vi "B7_72.vi"(4 "error in":T13, 7 "Command":T14) -> (0 "error out":T13, 3 "Response":T11)   [LabVIEW 2018]
uses:
  MOKO_LabViewLibrary/MokoLowLevel/MokoLowLovelControl/MLLC_Command.ctl
  MOKO_LabViewLibrary/MokoLowLevel/MokoLowLovelControl/MLLC_Error.ctl
  MOKO_LabViewLibrary/MokoLowLevel/MokoLowLovelControl/MLLC_Mode.ctl
  MOKO_LabViewLibrary/MokoLowLevel/MokoLowLovelControl/MLLC_Response.ctl
  MOKO_LabViewLibrary/MokoLowLevel/MokoLowLovelControl/MLLC_DriverName.ctl
  MOKO_LabViewLibrary/MokoLowLevel/MokoLowLovelControl/MLLC_ResponseInit.ctl
  MOKO_LabViewLibrary/MokoLowLevel/MokoLowLovelControl/MLLC_Request.ctl
  MOKO_LabViewLibrary/MokoLowLevel/MokoLowLovelControl/MLLC_ErrorCode.ctl
  MOKO_LabViewLibrary/MokoLowLevel/MokoLowLovelControl/MLLC_ConnectCluster.ctl
  MOKO_LabViewLibrary/MokoLowLevel/MokoLowLovelControl/MLLC_InterfaceType.ctl
  MOKO_LabViewLibrary/MokoLowLevel/MokoLowLovelControl/MLLC_OpenedSession.ctl
  MOKO_LabViewLibrary/MokoLowLevel/MokoLowLovelControl/MLLC_InterfaceSettings.ctl
  MOKO_LabViewLibrary/MokoLowLevel/MokoLowLovelControl/MLLC_InterfaceKind.ctl
  MOKO_LabViewLibrary/MokoLowLevel/MokoLowLovelControl/MLLC_Rs232Settings.ctl
panel:
  in  "Settings":T7={"Data"={"Connect"={"InterfaceType"=enum."VISA", "OpenedSession"="COM1", "InterfaceSettings"={"Interface"=enum."RS232", "EOS 4 read"=enum."LF (\\n)", "EOS 4 write"=enum."LF (\\n)", "TMO, ms"=10000, "Sett"=variant(cluster{"Baud Rate":u32, "Data Bits":u16, "Parity":u16, "Stop Bits":u16, "Flow Control":u16, "Eho":bool} {"Baud Rate"=75, "Data Bits"=0, "Parity"=0, "Stop Bits"=0, "Flow Control"=0, "Eho"=FALSE})}}, "Delay, ms"=100, "Function"=enum."VDC"}, "Saved Data"=variant}
  in  "Error Code":T6=5422
  in  "Request":T8="B2"
  in  "ResponseInit":T9="U4G1A0"
  in  "Driver Name":T10="B7_72"
  in  "Mode":T12=enum."Check"
  # "B7-72"
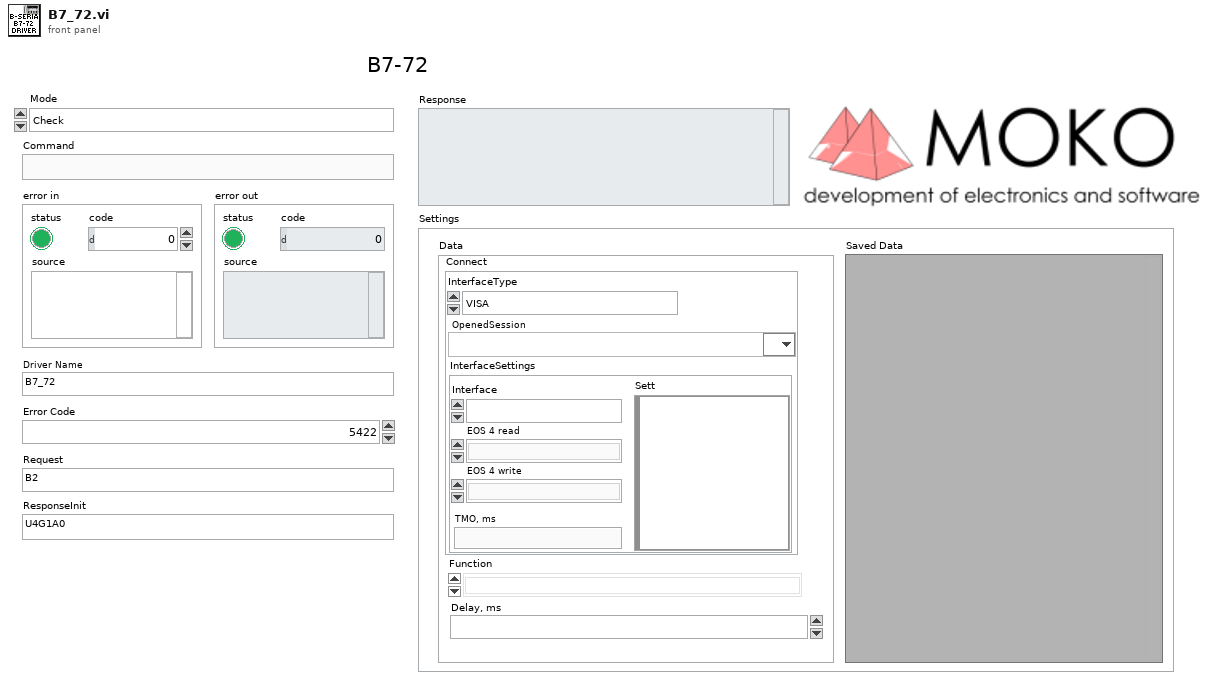
[diagram p1: front panel]
types:
  T1 = typedef "MLLC_ConnectCluster.ctl" = cluster{"InterfaceType":T2, "OpenedSession":T3, "InterfaceSettings":T4}
  T2 = typedef "MLLC_InterfaceType.ctl" = enum16{"VISA", "Prologix USB-GPIB"}
  T3 = typedef "MLLC_OpenedSession.ctl" = refnum<visa-resource-name>
  T4 = typedef "MLLC_InterfaceSettings.ctl" = cluster{"Interface":T5, "EOS 4 read":enum16{"Default (=EOS 4 write)", "CR (\\r)", "LF (\\n)", "None"}, "EOS 4 write":enum16{"CR+LF (\\r\\n)", "CR (\\r)", "LF (\\n)", "None"}, "TMO, ms":i32, "Sett":variant}
  T5 = typedef "MLLC_InterfaceKind.ctl" = enum16{"RS232", "GPIB", "USB", "Ethernet", "another"}
  T6 = typedef "MLLC_ErrorCode.ctl" = u32
  T7 = cluster{"Data":cluster{"Connect":T1, "Delay, ms":T6, "Function":enum16{"F", "T", "R4", "R", "IAC", "IDC", "VAC", "VDC"}}, "Saved Data":variant}
  T8 = typedef "MLLC_Request.ctl" = string
  T9 = typedef "MLLC_ResponseInit.ctl" = string
  T10 = typedef "MLLC_DriverName.ctl" = string
  T11 = typedef "MLLC_Response.ctl" = string
  T12 = typedef "MLLC_Mode.ctl" = enum16{"get", "set", "close", "Init", "Check"}
  T13 = typedef "MLLC_Error.ctl" = errorcluster
  T14 = typedef "MLLC_Command.ctl" = string
  T15 = cluster{"Connect":T1, "Delay, ms":T6, "Function":enum16{"F", "T", "R4", "R", "IAC", "IDC", "VAC", "VDC"}}
  T16 = enum16{"F", "T", "R4", "R", "IAC", "IDC", "VAC", "VDC"}
  T17 = typedef "MLLC_Rs232Settings.ctl" = cluster{"Baud Rate":u32, "Data Bits":u16, "Parity":u16, "Stop Bits":u16, "Flow Control":u16, "Eho":bool, "Address":dbl}
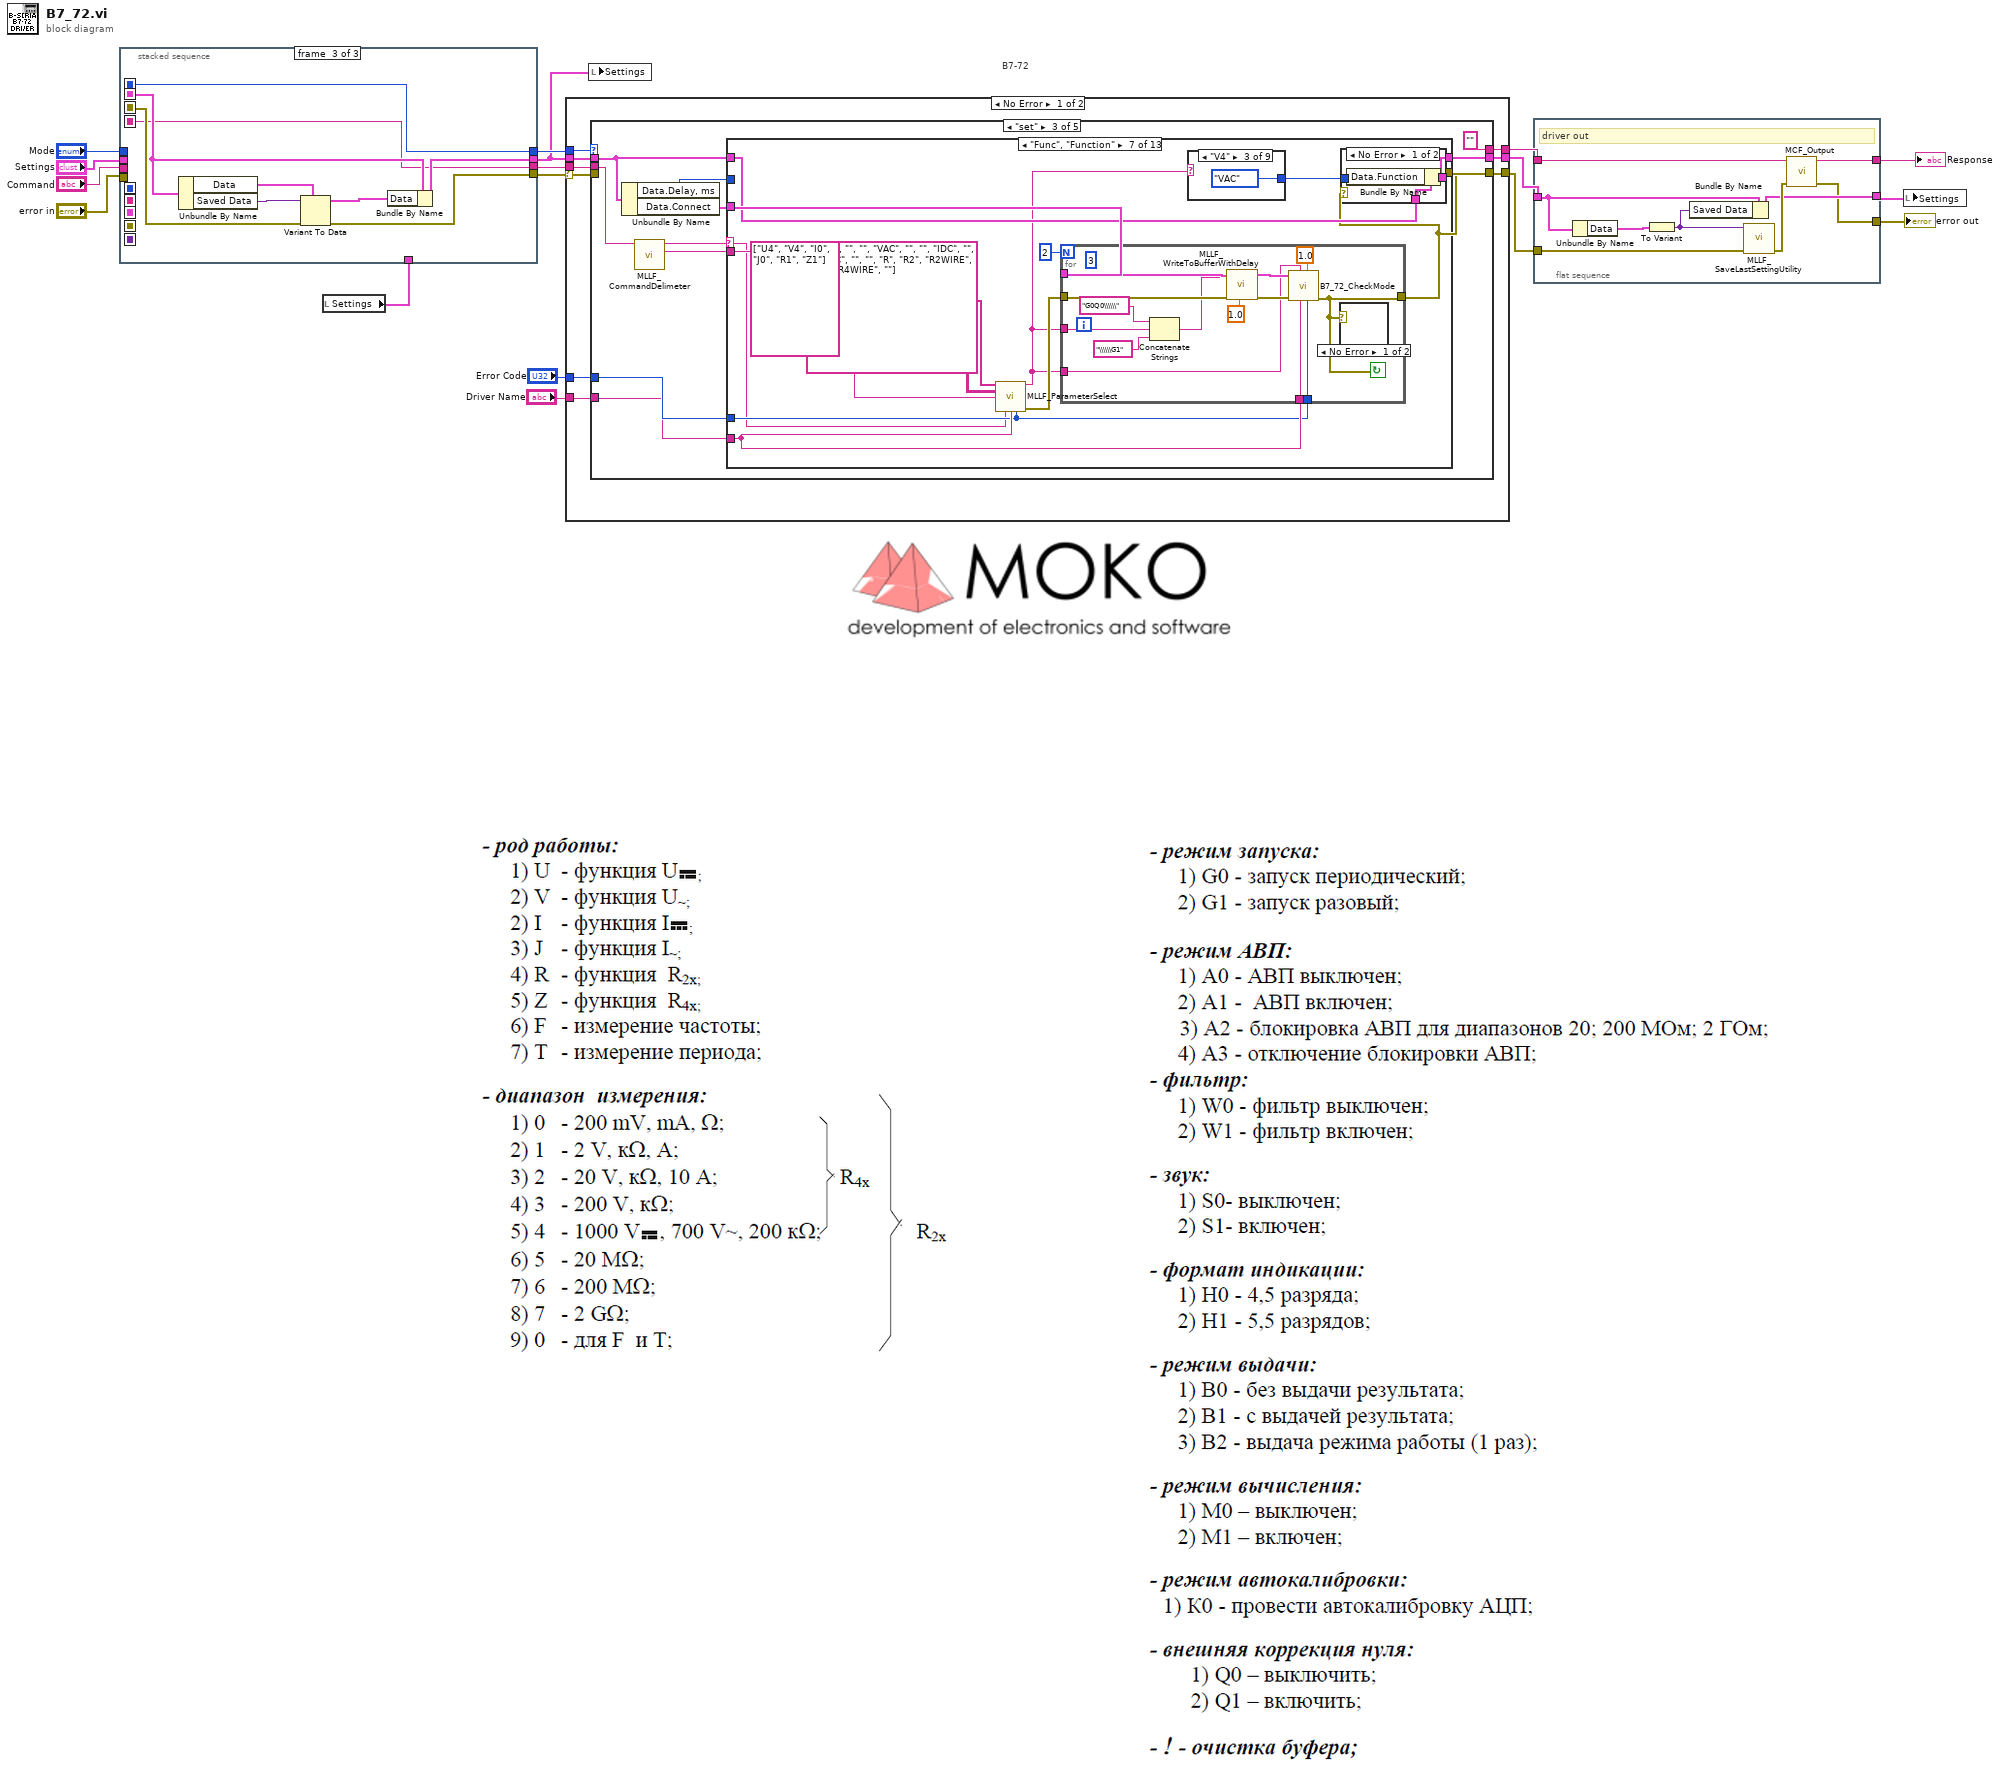
[diagram p0: block diagram]
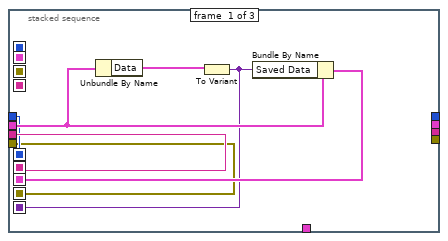
[diagram p2: hidden frame]
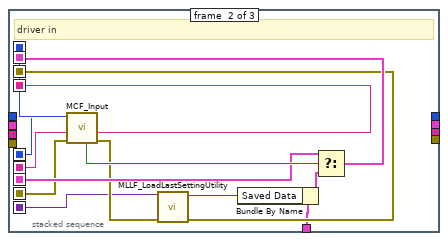
[diagram p3: hidden frame]
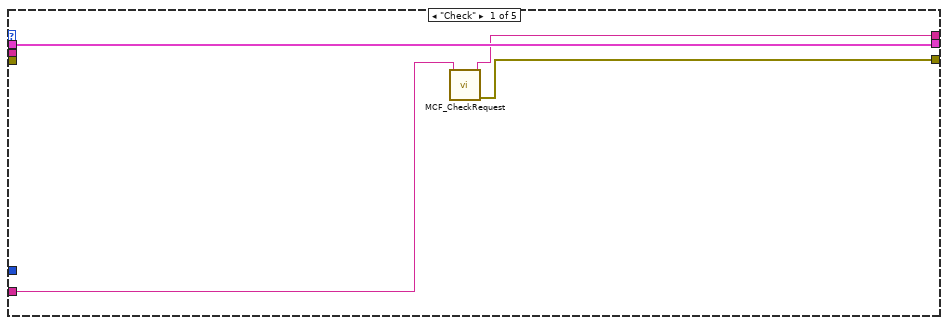
[diagram p4: hidden frame]
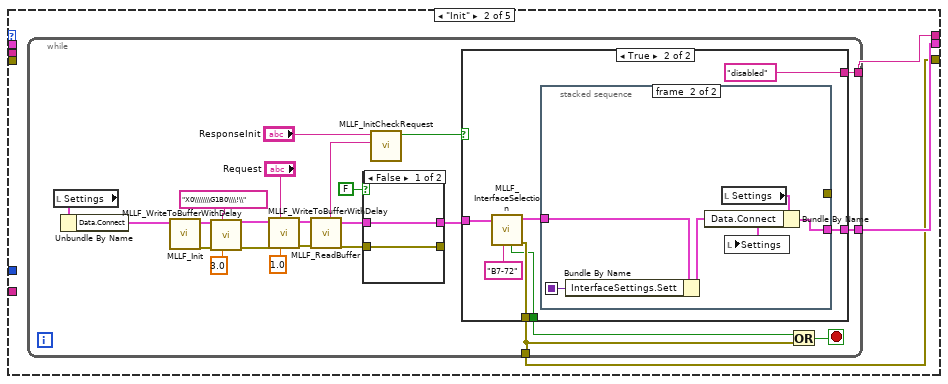
[diagram p5: hidden frame]
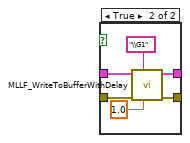
[diagram p6: hidden frame]
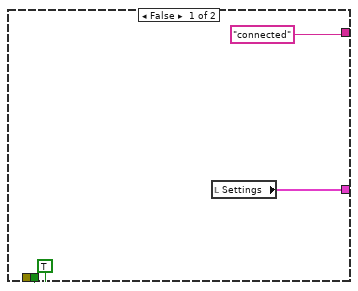
[diagram p7: hidden frame]
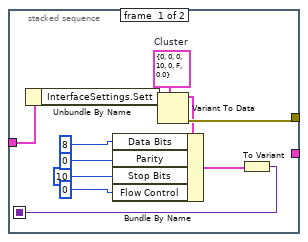
[diagram p8: hidden frame]
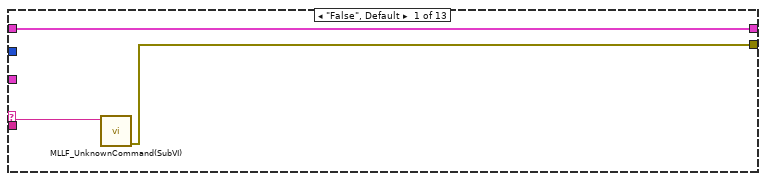
[diagram p9: hidden frame]
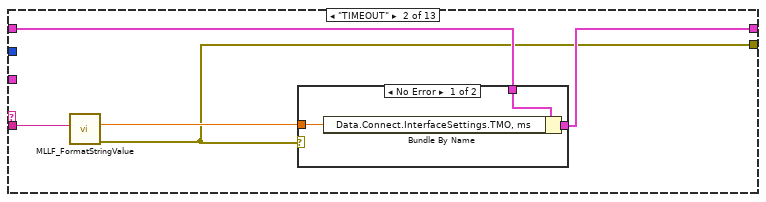
[diagram p10: hidden frame]
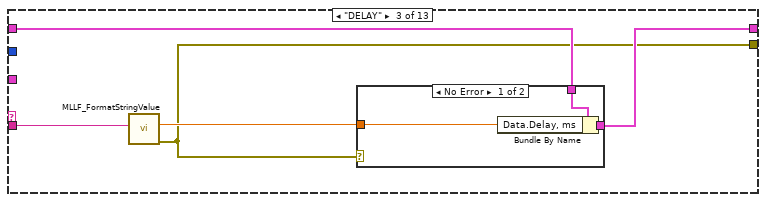
[diagram p12: hidden frame]
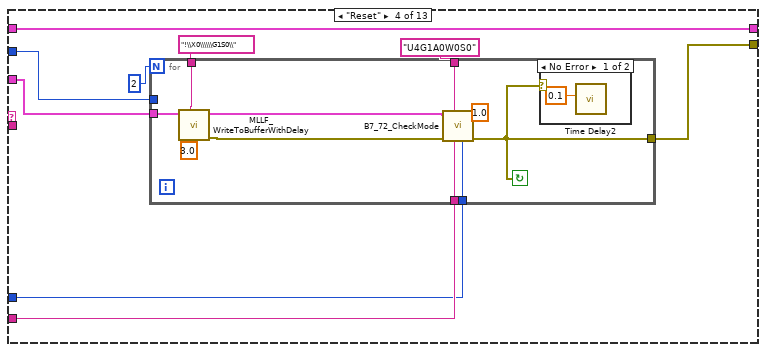
[diagram p14: hidden frame]
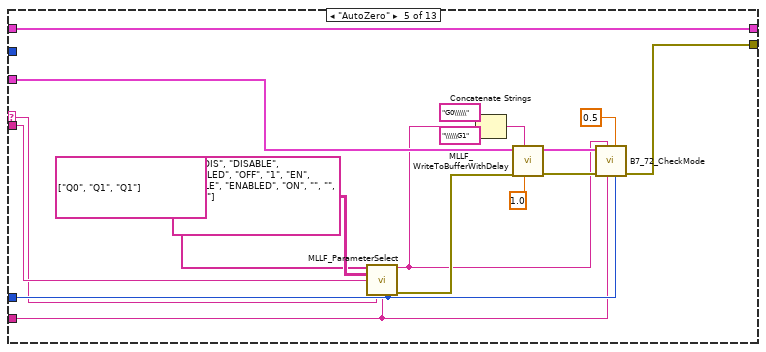
[diagram p16: hidden frame]
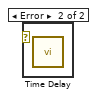
[diagram p18: hidden frame]
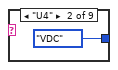
[diagram p20: hidden frame]
diagram:
  # "B7-72"
  n1 = local read "Settings"() -> (w11:T7)
  n2 = stacked-sequence {
    seq-local: [w20 _ _] -> [_ w36 _]
    seq-local: [w19 _ _] -> [_ w37 _]
    seq-local: [w22 _ _] -> [_ w32 _]
    seq-local: [w18 _ _] -> [_ w31 _]
    seq-local: [w21 _ _] -> [_ w27 _]
    seq-local: [_ w28 _] -> [_ _ w44]
    seq-local: [_ w38 _] -> [_ _ w41]
    seq-local: [_ w35 _] -> [_ _ w40]
    seq-local: [_ w34 _] -> [_ _ w45]
    tunnel: "Command" -> [w20 _ _]
    tunnel: "Mode" -> [w19 _ _]
    tunnel: "error in" -> [w18 _ _]
    tunnel: "Settings" -> [w23 _ _]
    tunnel: w11 -> [_ w26 _]
    tunnel: [_ _ w40] -> w8
    tunnel: [_ _ w43] -> w9
    tunnel: [_ _ w42] -> w7
    tunnel: [_ _ w41] -> w10
    frame #0 {
      n3 = Unbundle By Name(w23) -> ("Data"=w24:T15)
      n4 = To Variant(anything=w24) -> (Variant=w21:variant)
      n5 = Bundle By Name(cluster=w23, "Saved Data"=w21) -> (w22:T7)
    }
    frame #1 {
      # "driver in"
      n6 = call "MCF_Input.vi"("Error In"=w31, "Command in"=w36, "Mode in"=w37) -> ("Error Out"=w30:errorcluster, "Command out"=w35:string, "Mode out"=w38:T12, "Boolean"=w33:bool)  [unwired: 5 in]
      n7 = call "MLLF_LoadLastSettingUtility.vi"("Error In"=w30, "Save data in"=w27) -> ("Error Out"=w28:errorcluster, "Save data out"=w25:variant)  [unwired: 8 in]
      n8 = Bundle By Name(cluster=w26, "Saved Data"=w25) -> (w29:T7)
      n9 = Select(t=w32, s=w33, f=w29) -> (s? t:f=w34:T7)
    }
    frame #2 {
      n10 = Unbundle By Name(w45) -> ("Data"=w46:T15, "Saved Data"=w39:variant)
      n11 = Variant To Data(error in=w44, type=w46, Variant=w39) -> (data=w47:T15, error out=w42:errorcluster)
      n12 = Bundle By Name(cluster=w45, "Data"=w47) -> (w43:T7)
    }
  }
  n13 = case shown="No Error" w7 {
    selector: w7 -> [w54 w452]
    tunnel: w10 -> [w56 _]
    tunnel: w8 -> [w55 _]
    tunnel: w9 -> [w51 w451]
    tunnel: "Error Code" -> [w53 _]
    tunnel: "Driver Name" -> [w52 _]
    tunnel: [w50 "" ("String")] -> w6
    tunnel: [w49 w451] -> w5
    tunnel: [w48 w452] -> w4
    frame No Error {
      n14 = case shown="\"set\"" w56 {
        tunnel: [w59 w63 "" ("String") w385 "" ("String")] -> w50
        tunnel: [w58 w61 w122 w384 w448] -> w48
        tunnel: w55 -> [_ _ w132 w397 _]
        tunnel: w54 -> [_ _ _ _ _]
        tunnel: w53 -> [_ _ w131 w394 _]
        tunnel: w52 -> [w57 _ w128 w393 _]
        tunnel: w51 -> [w60 _ w130 w396 w447]
        tunnel: [w60 w62 w129 w395 w447] -> w49
        frame "Check" {
          n15 = call "MCF_CheckRequest.vi"("Driver Name"=w57) -> ("Error Out"=w58:errorcluster, "Output String"=w59:string)  [unwired: 9 in]
        }
        frame "Init" {
          n16 = while {
            tunnel: [w79] -> w61
            tunnel: [w65] -> w62
            tunnel: [w64] -> w63
            stop <- w78 stop-if-true
            n17 = local read "Settings"() -> (w87:T7)
            n18 = Unbundle By Name(w87) -> ("Data.Connect"=w83:T1)
            n19 = call "MLLF_Init.vi"("DriverConnect in"=w83) -> ("Error Out"=w72:errorcluster, "DriverConnect out"=w73:T1)  [unwired: 7 in]
            n20 = call "MLLF_WriteToBufferWithDelay.vi"("Delay Time ( 0,05 s)"=3.0 ("Delay Time (s)"), "Command"="X0\\\\\\\\G1B0\\\\!\\" ("String"), "Error In"=w72, "DriverConnect in"=w73) -> ("Error Out"=w76:errorcluster, "DriverConnect out"=w75:T1)  [unwired: 6 in]
            n21 = call "MLLF_WriteToBufferWithDelay.vi"("Delay Time ( 0,05 s)"=1.0 ("Delay Time (s)"), "Command"="Request", "Error In"=w76, "DriverConnect in"=w75) -> ("Error Out"=w85:errorcluster, "DriverConnect out"=w86:T1)  [unwired: 6 in]
            n22 = call "MLLF_ReadBuffer.vi"("Error In"=w85, "DriverConnect in"=w86) -> ("Error Out"=w80:errorcluster, "DriverConnect out"=w81:T1, "String"=w67:string)  [unwired: 6 in]
            n23 = case shown="False" FALSE {
              tunnel: [w88 w94] -> _
              tunnel: [w89 w93] -> w82
              tunnel: w81 -> [w89 w92]
              tunnel: w80 -> [w88 w91]
              frame False {
              }
              frame True {
                n24 = call "MLLF_WriteToBufferWithDelay.vi"("Delay Time ( 0,05 s)"=1.0 ("Delay Time (s)"), "Command"="\\G1" ("String"), "Error In"=w91, "DriverConnect in"=w92) -> ("Error Out"=w94:errorcluster, "DriverConnect out"=w93:T1)  [unwired: 6 in]
              }
            }
            n25 = call "MLLF_InitCheckRequest.vi"("Answer"=w67, "Response Init"="ResponseInit") -> ("Design"=w66:bool)  [unwired: 6 in, 3 out]
            n26 = case shown="True" w66 {
              tunnel: w82 -> [_ w105]
              tunnel: [_ w102] -> w79
              tunnel: [TRUE w99] -> w77
              tunnel: [w96 w101] -> w65
              tunnel: ["connected" "disabled"] -> w64
              frame False {
                n27 = local read "Settings"() -> (w96:T7)
              }
              frame True {
                n28 = call "MLLF_InterfaceSelection.vi"("Driver Name"="B7-72" ("String"), "DriverConnect in"=w105) -> ("error out"=w102:T13, "DriverConnect out"=w103:T1, "stop init?"=w99:bool)  [unwired: 5 in, 2 out]
                n29 = stacked-sequence {
                  seq-local: [w107 _] -> [_ w120]
                  tunnel: w103 -> [w106 w118]
                  tunnel: [w114 _] -> _
                  tunnel: [_ w119] -> w101
                  frame #0 {
                    w115 = T17 {"Baud Rate"=0, "Data Bits"=0, "Parity"=0, "Stop Bits"=10, "Flow Control"=0, "Eho"=FALSE, "Address"=0.0}  # Cluster
                    n30 = Unbundle By Name(w106) -> ("InterfaceSettings.Sett"=w116:variant)
                    n31 = Variant To Data(type=w115, Variant=w116) -> (data=w113:T17, error out=w114:errorcluster)  [unwired: 1 in]
                    n32 = Bundle By Name(cluster=w113, "Data Bits"=u16 8 ("Serial Settings:Data Bits"), "Parity"=u16 0 ("Serial Settings:Parity"), "Stop Bits"=u16 10 ("Serial Settings:Stop Bits"), "Flow Control"=u16 0 ("Serial Settings:Flow Control")) -> (w108:T17)
                    n33 = To Variant(anything=w108) -> (Variant=w107:variant)
                  }
                  frame #1 {
                    n34 = Bundle By Name(cluster=w118, "InterfaceSettings.Sett"=w120) -> (w117:T1)
                    n35 = local read "Settings"() -> (w121:T7)
                    n36 = Bundle By Name(cluster=w121, "Data.Connect"=w117) -> (w119:T7)
                    n37 = local write "Settings"(w119) -> ()
                  }
                }
              }
            }
            n38 = Or(x=w77, y=w79) -> (x .or. y?=w78:bool)
          }
        }
        frame "set" {
          n39 = Unbundle By Name(w130) -> ("Data.Delay, ms"=w125:T6, "Data.Connect"=w126:T1)
          n40 = call "MLLF_CommandDelimeter.vi"("command with param"=w132) -> ("param 1"=w123:string, "command"=w124:string)  [unwired: 6 in, 3 out]
          n41 = case shown="\"Func\", \"Function\"" w124 {
            selector: w124 -> [w134 _ _ _ w174 _ w193 _ _ w276 w305 w330 w355]
            tunnel: w123 -> [_ w138 w147 _ w186 _ w205 w233 _ w285 w314 w338 w364]
            tunnel: [w133 w136 w145 w159 w183 _ w196 w237 _ w283 w306 w331 w358] -> w122
            tunnel: w131 -> [_ _ _ w157 w188 _ w199 w239 _ w282 w307 w333 w359]
            tunnel: w130 -> [w135 w139 w148 w155 w191 w192 w198 w244 w275 w288 w316 w341 w367]
            tunnel: [w135 w140 w149 w155 w191 w192 w203 w244 w275 w288 w316 w341 w367] -> w129
            tunnel: w126 -> [_ _ _ w156 w181 _ w201 w241 _ w280 w311 w336 w362]
            tunnel: w128 -> [_ _ _ w158 w187 _ w200 w238 _ w281 w308 w332 w360]
            tunnel: w125 -> [_ _ _ w154 _ _ _ _ _ w277 _ _ w356]
            frame "False", Default {
              n42 = call "MLLF_UnknownCommand(SubVI).vi"("Unknown command"=w134) -> ("error out"=w133:errorcluster)  [unwired: 10 in]
            }
            frame "TIMEOUT" {
              n43 = call "MLLF_FormatStringValue.vi"("String Value"=w138) -> ("error out"=w136:T13, "number"=w137:dbl)  [unwired: 8 in, 1 out]
              n44 = case shown="No Error" w136 {
                tunnel: [w143 w144] -> w140
                tunnel: w139 -> [w142 w144]
                tunnel: w137 -> [w141 _]
                frame No Error {
                  n45 = Bundle By Name(cluster=w142, "Data.Connect.InterfaceSettings.TMO, ms"=w141) -> (w143:T7)
                }
                frame Error {
                }
              }
            }
            frame "DELAY" {
              n46 = call "MLLF_FormatStringValue.vi"("String Value"=w147) -> ("error out"=w145:T13, "number"=w146:dbl)  [unwired: 8 in, 1 out]
              n47 = case shown="No Error" w145 {
                tunnel: [w152 w153] -> w149
                tunnel: w148 -> [w151 w153]
                tunnel: w146 -> [w150 _]
                frame No Error {
                  n48 = Bundle By Name(cluster=w151, "Data.Delay, ms"=w150) -> (w152:T7)
                }
                frame Error {
                }
              }
            }
            frame "Reset" {
              n49 = for {
                N: 2 -> [_]
                tunnel: w156 -> [w172]
                tunnel: w158 -> [w170]
                tunnel: w157 -> [w169]
                tunnel: [w163] -> w159
                tunnel: "!\\X0\\\\\\G1S0\\" ("String") -> [w168]
                tunnel: "U4G1A0W0S0" ("Mode2check") -> [w165]
                tunnel: w154 -> [_]
                stop <- w163 continue-if-true
                n50 = call "MLLF_WriteToBufferWithDelay.vi"("Delay Time ( 0,05 s)"=3.0 ("Delay Time (s)"), "Command"=w168, "DriverConnect in"=w172) -> ("Error Out"=w164:errorcluster, "DriverConnect out"=w171:T1)  [unwired: 7 in]
                n51 = call "B7_72_CheckMode.vi"("Error Code"=w169, "Delay Time (s)"=1.0, "Driver Name"=w170, "Mode2check"=w165, "error in"=w164, "DriverConnect in"=w171) -> ("error out"=w163:T13)  [unwired: 4 in, 1 out]
                n52 = case shown="No Error" w163 {
                  frame No Error {
                    n53 = call "Time Delay2"("Delay Time (s)"=0.1) -> ()  [unwired: 10 in, 1 out]
                  }
                  frame Error {
                  }
                }
              }
            }
            frame "AutoZero" {
              n54 = call "MLLF_ParameterSelect.vi"("Command to equipment"=string[] ["Q0", "Q1", "Q1"] ("Names"), "Names"=string[][] [["0", "DIS", "DISABLE", "DISABLED", "OFF"], ["1", "EN", "ENABLE", "ENABLED", "ON"], ["", "", "", "", ""]], "Input"=w186, "Command"=w174, "Driver Name"=w187, "Error Code"=w188) -> ("Choice"=w179:string, "Error Out"=w180:errorcluster)  [unwired: 8 in]
              n55 = Concatenate Strings("G0\\\\\\" ("string"), w179, "\\\\\\G1" ("string")) -> (w178:string)
              n56 = call "MLLF_WriteToBufferWithDelay.vi"("Delay Time ( 0,05 s)"=1.0 ("Delay Time (s)"), "Command"=w178, "Error In"=w180, "DriverConnect in"=w181) -> ("Error Out"=w182:errorcluster, "DriverConnect out"=w185:T1)  [unwired: 6 in]
              n57 = call "B7_72_CheckMode.vi"("Error Code"=w188, "Delay Time (s)"=0.5, "Driver Name"=w187, "Mode2check"=w179, "error in"=w182, "DriverConnect in"=w185) -> ("error out"=w183:T13)  [unwired: 4 in, 1 out]
            }
            frame "--------------------Main----------------------" {
            }
            frame "Func", "Function" {
              n58 = call "MLLF_ParameterSelect.vi"("Command to equipment"=string[] ["U4", "V4", "I0", "J0", "R1", "Z1"] ("Names"), "Names"=string[][] [["VDC", "", ""], ["VAC", "", ""], ["IDC", "", ""], ["IAC", "", ""], ["R", "R2", "R2WIRE"], ["R4", "R4WIRE", ""]], "Input"=w205, "Command"=w193, "Driver Name"=w200, "Error Code"=w199) -> ("Choice"=w194:string, "Error Out"=w197:errorcluster)  [unwired: 8 in]
              n59 = for {
                N: 2 -> [_]
                tunnel: w201 -> [w220]
                tunnel: w200 -> [w216]
                tunnel: w199 -> [w215]
                tunnel: w197 -> [w219]
                tunnel: [w213] -> w196
                tunnel: w194 -> [w211]
                tunnel: w194 -> [w212]
                stop <- w213 continue-if-true
                (unwired) 3
                n60 = Concatenate Strings("G0Q0\\\\\\" ("string"), w212, "\\\\\\G1" ("string")) -> (w209:string)
                n61 = call "MLLF_WriteToBufferWithDelay.vi"("Delay Time ( 0,05 s)"=1.0 ("Delay Time (s)"), "Command"=w209, "Error In"=w219, "DriverConnect in"=w220) -> ("Error Out"=w214:errorcluster, "DriverConnect out"=w218:T1)  [unwired: 6 in]
                n62 = call "B7_72_CheckMode.vi"("Error Code"=w215, "Delay Time (s)"=1.0, "Driver Name"=w216, "Mode2check"=w211, "error in"=w214, "DriverConnect in"=w218) -> ("error out"=w213:T13)  [unwired: 4 in, 1 out]
                n63 = case shown="No Error" w213 {
                  frame No Error {
                  }
                  frame Error {
                    n64 = call "Time Delay"() -> ()  [unwired: 11 in, 1 out]
                  }
                }
              }
              n65 = case shown="\"V4\"" w194 {
                tunnel: [_ T16."VDC" ("Function") T16."VAC" ("Function") T16."IDC" ("Function") T16."IAC" ("Function") T16."R" ("Function") T16."R4" ("Function") T16."F" ("Function") T16."T" ("Function")] -> w202
                frame "False", Default {
                }
                frame "U4" {
                }
                frame "V4" {
                }
                frame "I0" {
                }
                frame "J0" {
                }
                frame "R1" {
                }
                frame "Z1" {
                }
                frame "F0" {
                }
                frame "T0" {
                }
              }
              n66 = case shown="No Error" w196 {
                tunnel: [w231 w232] -> w203
                tunnel: w198 -> [w230 w232]
                tunnel: w202 -> [w229 _]
                frame No Error {
                  n67 = Bundle By Name(cluster=w230, "Data.Function"=w229) -> (w231:T7)
                }
                frame Error {
                }
              }
            }
            frame "RANGE" {
              n68 = Unbundle By Name(w244) -> ("Data.Function"=w245:T16)
              n69 = Index Array(array=string[] ["F", "T", "Z", "R", "J", "I", "V", "U"] ("Names"), index=w245) -> (element=w243:string)
              n70 = case shown="\"1\", Default" w233 {
                selector: w233 -> [w259 _]
                tunnel: [w260 _] -> w240
                tunnel: [w263 "1A1" ("String")] -> w242
                tunnel: w243 -> [w264 _]
                frame "1", Default {
                  n71 = call "MLLF_FormatStringValue.vi"("String Value"=w259) -> ("error out"=w260:T13, "number"=w262:dbl)  [unwired: 8 in, 1 out]
                  n72 = case shown="\"R\", \"Z\"" w264 {
                    tunnel: [w265 w272 "0" ("R/O")] -> w263
                    tunnel: w262 -> [w266 w269 _]
                    tunnel: string[] ["0", "1", "2", "3", "4", "5", "6", "7"] ("RangeCommand") -> [w268 w271 _]
                    frame "R", "Z" {
                      n73 = call "B7_72_82_StandartRangeSelect (SubVI).vi"("Control Point"=w266, "RangeDigit"=dbl[] [200.0, 2000.0, 20000.0, 200000.0, 2000000.0, 20000000.0, 200000000.0, 2000000000.0], "RangeCommand"=w268) -> ("R/O"=w265:string)  [unwired: 1 in]
                    }
                    frame "U", "V", Default {
                      n74 = call "B7_72_82_StandartRangeSelect (SubVI).vi"("Control Point"=w269, "RangeDigit"=dbl[] [0.2, 2.0, 20.0, 200.0, 1000.0], "RangeCommand"=w271) -> ("R/O"=w272:string)  [unwired: 1 in]
                    }
                    frame "I", "J" {
                    }
                  }
                }
                frame "auto" {
                }
              }
              n75 = Concatenate Strings(w243, w242) -> (w236:string)
              n76 = for {
                N: 2 -> [_]
                tunnel: w241 -> [w251]
                tunnel: w238 -> [w257]
                tunnel: w239 -> [w256]
                tunnel: w240 -> [w252]
                tunnel: [w255] -> w237
                tunnel: w236 -> [w248]
                stop <- w255 continue-if-true
                n77 = Concatenate Strings("G0Q0\\\\\\" ("string"), w248, "\\\\\\G1" ("string")) -> (w249:string)
                n78 = call "MLLF_WriteToBufferWithDelay.vi"("Delay Time ( 0,05 s)"=1.0 ("Delay Time (s)"), "Command"=w249, "Error In"=w252, "DriverConnect in"=w251) -> ("Error Out"=w253:errorcluster, "DriverConnect out"=w254:T1)  [unwired: 6 in]
                n79 = call "B7_72_CheckMode.vi"("Error Code"=w256, "Delay Time (s)"=0.5, "Driver Name"=w257, "Mode2check"=w248, "error in"=w253, "DriverConnect in"=w254) -> ("error out"=w255:T13)  [unwired: 4 in, 1 out]
                n80 = case shown="Error" w255 {
                  frame No Error {
                  }
                  frame Error {
                    n81 = call "Time Delay6"() -> ()  [unwired: 11 in, 1 out]
                  }
                }
              }
            }
            frame "-------------Supplemental------------" {
            }
            frame "ACQ", "ACQUISITION" {
              # "В этой функции большого смысла нет!"
              n82 = call "MLLF_ParameterSelect.vi"("Command to equipment"=string[] ["G0", "G1"] ("Names"), "Names"=string[][] [["CONT", "CONTINUOUS", ""], ["ONCE", "ONETIME", "1"]], "Input"=w285, "Command"=w276, "Driver Name"=w281, "Error Code"=w282) -> ("Choice"=w279:string, "Error Out"=w278:errorcluster)  [unwired: 8 in]
              n83 = for {
                N: 2 -> [_]
                tunnel: w280 -> [w304]
                tunnel: w282 -> [w302]
                tunnel: w281 -> [w301]
                tunnel: [w298] -> w283
                tunnel: w278 -> [w299]
                tunnel: w279 -> [w289]
                tunnel: w277 -> [w291]
                stop <- w298 continue-if-true
                n84 = Concatenate Strings(w289) -> (w290:string)
                n85 = call "MLLF_WriteToBufferWithDelay.vi"("Delay Time ( 0,05 s)"=3.0 ("Delay Time (s)"), "Command"=w290, "Error In"=w299, "DriverConnect in"=w304) -> ("Error Out"=w292:errorcluster, "DriverConnect out"=w303:T1)  [unwired: 6 in]
                n86 = Divide(x=w291, y=1000) -> (x/y=w294:dbl)
                n87 = call "Time Delay5"("error in (no error)"=w292, "Delay Time (s)"=w294) -> ("error out"=w293:errorcluster)  [unwired: 9 in]
                n88 = Wait (ms)(milliseconds to wait=u32 100) -> ()  [unwired: 1 out]
                n89 = call "B7_72_CheckMode.vi"("Error Code"=w302, "Delay Time (s)"=0.5, "Driver Name"=w301, "Mode2check"=w289, "error in"=w293, "DriverConnect in"=w303) -> ("error out"=w298:T13)  [unwired: 4 in, 1 out]
              }
            }
            frame "Filter" {
              n90 = call "MLLF_ParameterSelect.vi"("Command to equipment"=string[] ["W0", "W1"] ("Names"), "Names"=string[][] [["0", "DIS", "DISABLED", "DISABLE", "OFF"], ["1", "EN", "ENABLE", "ENABLED", "ON"]], "Input"=w314, "Command"=w305, "Driver Name"=w308, "Error Code"=w307) -> ("Choice"=w309:string, "Error Out"=w310:errorcluster)  [unwired: 8 in]
              n91 = for {
                N: 2 -> [_]
                tunnel: w311 -> [w329]
                tunnel: w308 -> [w324]
                tunnel: w307 -> [w323]
                tunnel: [w321] -> w306
                tunnel: w310 -> [w318]
                tunnel: w309 -> [w317]
                stop <- w321 continue-if-true
                n92 = Concatenate Strings("G0Q0\\" ("string"), w317, "\\\\G1" ("string")) -> (w328:string)
                n93 = call "MLLF_WriteToBufferWithDelay.vi"("Delay Time ( 0,05 s)"=1.0 ("Delay Time (s)"), "Command"=w328, "Error In"=w318, "DriverConnect in"=w329) -> ("Error Out"=w322:errorcluster, "DriverConnect out"=w327:T1)  [unwired: 6 in]
                n94 = call "B7_72_CheckMode.vi"("Error Code"=w323, "Delay Time (s)"=0.5, "Driver Name"=w324, "Mode2check"=w317, "error in"=w322, "DriverConnect in"=w327) -> ("error out"=w321:T13)  [unwired: 4 in, 1 out]
                n95 = case shown="Error" w321 {
                  frame No Error {
                  }
                  frame Error {
                    n96 = call "Time Delay3"() -> ()  [unwired: 11 in, 1 out]
                  }
                }
              }
            }
            frame "DIGITS", "DISP", "DISPLAY", "INTEGRATIONTIME", "INTTIME" {
              n97 = call "MLLF_ParameterSelect.vi"("Command to equipment"=string[] ["H1", "H0"] ("Names"), "Names"=string[][] [["6.5", "6,5", "7"], ["5.5", "5,5", "6"]], "Input"=w338, "Command"=w330, "Driver Name"=w332, "Error Code"=w333) -> ("Choice"=w334:string, "Error Out"=w335:errorcluster)  [unwired: 8 in]
              n98 = for {
                N: 2 -> [_]
                tunnel: w336 -> [w354]
                tunnel: w332 -> [w349]
                tunnel: w333 -> [w348]
                tunnel: [w346] -> w331
                tunnel: w335 -> [w343]
                tunnel: w334 -> [w342]
                stop <- w346 continue-if-true
                n99 = Concatenate Strings("G0Q0\\" ("string"), w342, "\\\\G1" ("string")) -> (w353:string)
                n100 = call "MLLF_WriteToBufferWithDelay.vi"("Delay Time ( 0,05 s)"=1.0 ("Delay Time (s)"), "Command"=w353, "Error In"=w343, "DriverConnect in"=w354) -> ("Error Out"=w347:errorcluster, "DriverConnect out"=w352:T1)  [unwired: 6 in]
                n101 = call "B7_72_CheckMode.vi"("Error Code"=w348, "Delay Time (s)"=0.5, "Driver Name"=w349, "Mode2check"=w342, "error in"=w347, "DriverConnect in"=w352) -> ("error out"=w346:T13)  [unwired: 4 in, 1 out]
                n102 = case shown="Error" w346 {
                  frame No Error {
                  }
                  frame Error {
                    n103 = call "Time Delay4"() -> ()  [unwired: 11 in, 1 out]
                  }
                }
              }
            }
            frame "SND", "SOUND" {
              n104 = call "MLLF_ParameterSelect.vi"("Command to equipment"=string[] ["S0", "S1"] ("Names"), "Names"=string[][] [["0", "DIS", "DISABLED", "DISABLE", "OFF"], ["1", "EN", "ENABLE", "ENABLED", "ON"]], "Input"=w364, "Command"=w355, "Driver Name"=w360, "Error Code"=w359) -> ("Choice"=w361:string, "Error Out"=w357:errorcluster)  [unwired: 8 in]
              n105 = for {
                N: 2 -> [_]
                tunnel: w362 -> [w383]
                tunnel: w359 -> [w381]
                tunnel: w360 -> [w380]
                tunnel: [w378] -> w358
                tunnel: w361 -> [w368]
                tunnel: w357 -> [w377]
                tunnel: w356 -> [w372]
                stop <- w378 continue-if-true
                n106 = Concatenate Strings(w368) -> (w369:string)
                n107 = call "MLLF_WriteToBufferWithDelay.vi"("Delay Time ( 0,05 s)"=2.0 ("Delay Time (s)"), "Command"=w369, "Error In"=w377, "DriverConnect in"=w383) -> ("Error Out"=w373:errorcluster, "DriverConnect out"=w382:T1)  [unwired: 6 in]
                n108 = Divide(x=w372, y=1000) -> (x/y=w371:dbl)
                n109 = call "Time Delay8"("error in (no error)"=w373, "Delay Time (s)"=w371) -> ("error out"=w374:errorcluster)  [unwired: 9 in]
                n110 = Wait (ms)(milliseconds to wait=u32 100) -> ()  [unwired: 1 out]
                n111 = call "B7_72_CheckMode.vi"("Error Code"=w381, "Delay Time (s)"=0.5, "Driver Name"=w380, "Mode2check"=w368, "error in"=w374, "DriverConnect in"=w382) -> ("error out"=w378:T13)  [unwired: 4 in, 1 out]
              }
            }
          }
        }
        frame "get" {
          n112 = Unbundle By Name(w396) -> ("Data.Connect"=w390:T1, "Data.Function"=w388:T16)
          n113 = call "MLLF_CommandDelimeter.vi"("command with param"=w397) -> ("param 1"=w386:string, "command"=w387:string)  [unwired: 6 in, 3 out]
          n114 = case shown="\"TIMEOUT\"" w387 {
            selector: w387 -> [w399 _ _]
            tunnel: [w398 _ w408] -> w392
            tunnel: w394 -> [_ _ _]
            tunnel: [w402 w405 w412] -> w395
            tunnel: w396 -> [w402 w405 w412]
            tunnel: [w400 w403 w409] -> w391
            tunnel: w390 -> [_ _ w410]
            tunnel: w393 -> [_ _ _]
            tunnel: w386 -> [_ _ w411]
            tunnel: w388 -> [_ _ w406]
            frame "False", Default {
              n115 = call "MLLF_UnknownCommand(SubVI).vi"("Unknown command"=w399) -> ("error out"=w398:errorcluster)  [unwired: 10 in]
              n116 = Build Array(0 ("TimeOut")) -> (w400:i32[])
            }
            frame "TIMEOUT" {
              n117 = Unbundle By Name(w405) -> ("Data.Connect.InterfaceSettings.TMO, ms"=w404:i32)
              n118 = Build Array(w404) -> (w403:i32[])
            }
            frame "FETCH", "READ" {
              n119 = for {
                N: 3 -> [_]
                tunnel: w411 -> [w438]
                tunnel: w410 -> [w419]
                tunnel: [w413] -> w409
                tunnel: [w426] -> w408
                tunnel: w406 -> [_]
                stop <- w426 continue-if-true
                n120 = Decimal String To Number(string=w438) -> (number=w437:i32)  [unwired: 2 in, 1 out]
                n121 = call "MLLF_WriteToBufferWithDelay.vi"("Delay Time ( 0,05 s)"=2.0 ("Delay Time (s)"), "Command"="G0B1\\\\\\!" ("String"), "DriverConnect in"=w419) -> ("Error Out"=w423:errorcluster, "DriverConnect out"=w424:T1)  [unwired: 7 in]
                n122 = In Range and Coerce(upper limit=100, x=w437, lower limit=1) -> (coerced(x)=w418:i32)  [unwired: 1 out]
                n123 = call "MLLF_ClearBuffer.vi"("Timeout(default = 300 ms)"=u32 500 ("Timeout"), "Error In"=w423, "DriverConnect in"=w424) -> ("Error Out"=w420:errorcluster, "DriverConnect out"=w421:T1)  [unwired: 5 in, 1 out]
                n124 = Increment(x=w418) -> (x+1=w417:i32)
                n125 = for {
                  N: w417 -> [_]
                  tunnel: [w444] -> w414 mode=indexing
                  tunnel: [w443] -> w433
                  tunnel: [w441] -> w432
                  tunnel: w421 -> [w440]
                  tunnel: w420 -> [w439]
                  stop <- w443 stop-if-true
                  n126 = call "MLLF_ReadBuffer.vi"("Error In"=w439, "DriverConnect in"=w440) -> ("Error Out"=w443:errorcluster, "DriverConnect out"=w441:T1, "String"=w442:string)  [unwired: 6 in]
                  n127 = Fract/Exp String To Number(use system decimal point (T)=FALSE, string=w442) -> (number=w444:dbl)  [unwired: 2 in, 1 out]
                }
                n128 = call "MLLF_WriteToBufferWithDelay.vi"("Delay Time ( 0,05 s)"=0.5 ("Delay Time (s)"), "Command"="\\G1B0\\!" ("String"), "Error In"=w433, "DriverConnect in"=w432) -> ("Error Out"=w427:errorcluster, "DriverConnect out"=w428:T1)  [unwired: 6 in]
                n129 = Delete From Array(array=w414, length=1, index=0) -> (array with subset deleted=w413:dbl[])  [unwired: 1 out]
                n130 = call "MLLF_ClearBuffer.vi"("Timeout(default = 300 ms)"=u32 300 ("Timeout"), "Error In"=w427, "DriverConnect in"=w428) -> ("Error Out"=w426:errorcluster)  [unwired: 5 in, 2 out]
              }
            }
          }
          n131 = call "MLLF_FormatOutputValueWithUnits.vi"("Format"="%.;%^#_7e" ("format string"), "error in"=w392, "ValuesIn"=w391) -> ("error out"=w384:T13, "Result string"=w385:T14)  [unwired: 7 in]
        }
        frame "close" {
          n132 = Unbundle By Name(w447) -> ("Data.Connect.OpenedSession"=w449:T3)
          n133 = VISA Close(VISA resource name=w449) -> (error out=w448:errorcluster)  [unwired: 1 in]
        }
      }
    }
    frame Error {
    }
  }
  n134 = local write "Settings"(w9) -> ()
  n135 = flat-sequence {
    tunnel: [w461] -> w3
    tunnel: [w453] -> _
    tunnel: w6 -> [w460]
    tunnel: w4 -> [w459]
    tunnel: w5 -> [w455]
    tunnel: [w457] -> w2
    tunnel: [w453] -> w1
    frame #0 {
      # "driver out"
      n136 = Unbundle By Name(w455) -> ("Data"=w454:T15)
      n137 = To Variant(anything=w454) -> (Variant=w456:variant)
      n138 = Bundle By Name(cluster=w455, "Saved Data"=w456) -> (w457:T7)
      n139 = call "MLLF_SaveLastSettingUtility.vi"("error in"=w459, "Saved Data"=w456) -> ("error out"=w458:T13)  [unwired: 8 in, 1 out]
      n140 = call "MCF_Output.vi"("Error In"=w458, "Input"=w460) -> ("Error Out"=w453:errorcluster, "Output"=w461:string)  [unwired: 8 in]
    }
  }
  n141 = local write "Settings"(w2) -> ()
  "error out" <- w1
  "Response" <- w3
